vi "Change Language.vi"(9 "Array IN":string[][](array[string]), 10 "References Pane":T1(array[cluster]), 11 "Langues/Languages":u8) -> ()   [LabVIEW 2013]
doc: "Jean-Marc Simard \nExaprom inc. 2009"
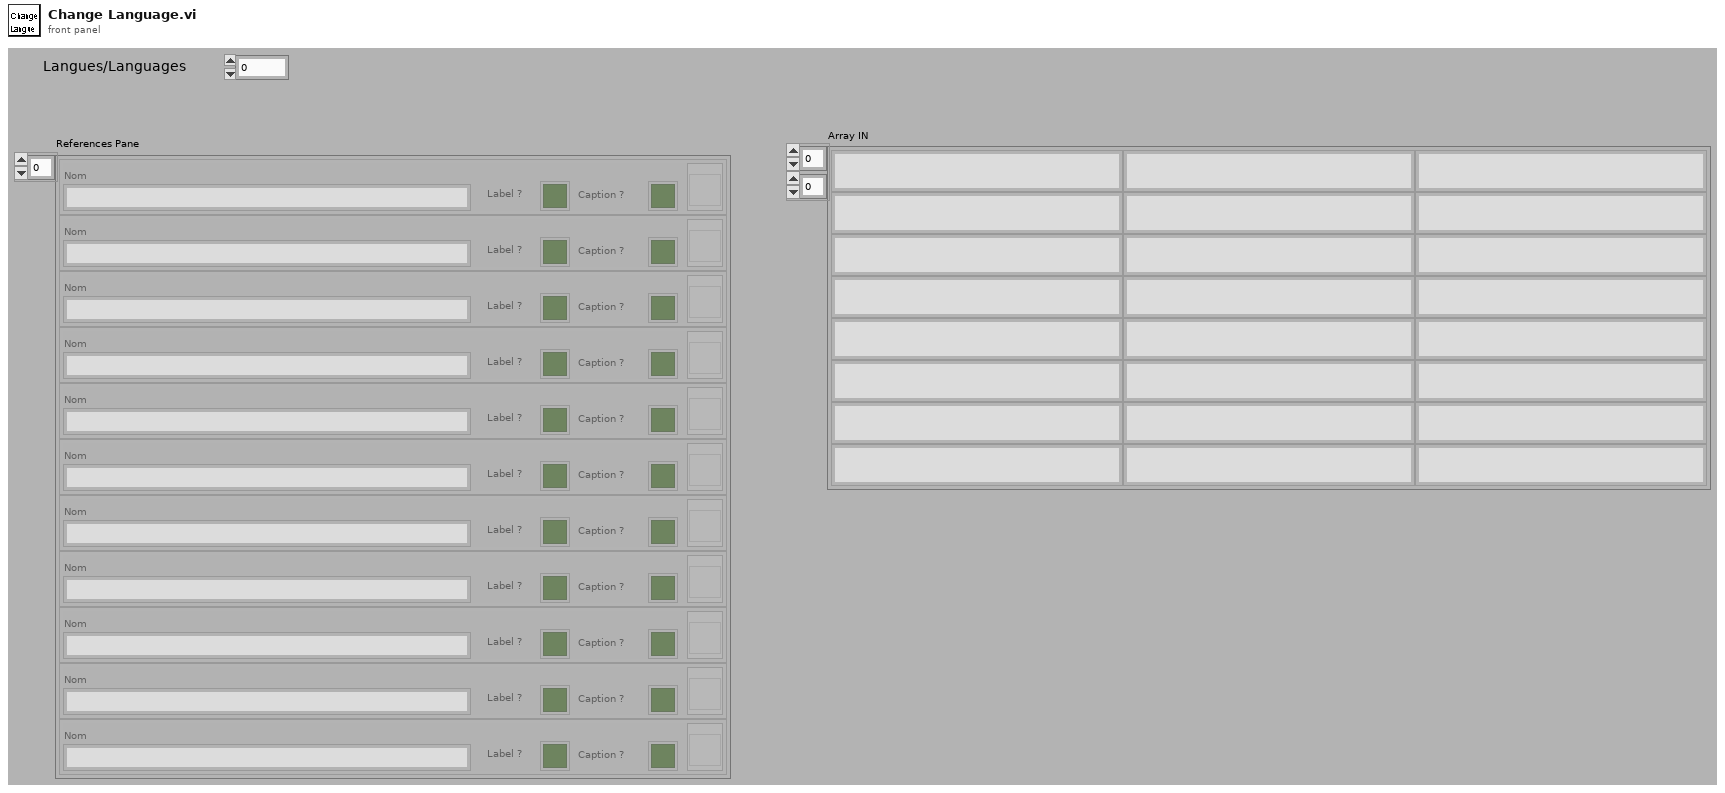
[diagram p1: front panel]
types:
  T1 = cluster{"Nom":string, "Label ?":bool, "Caption ?":bool, "Ref":refnum<vi>}[]
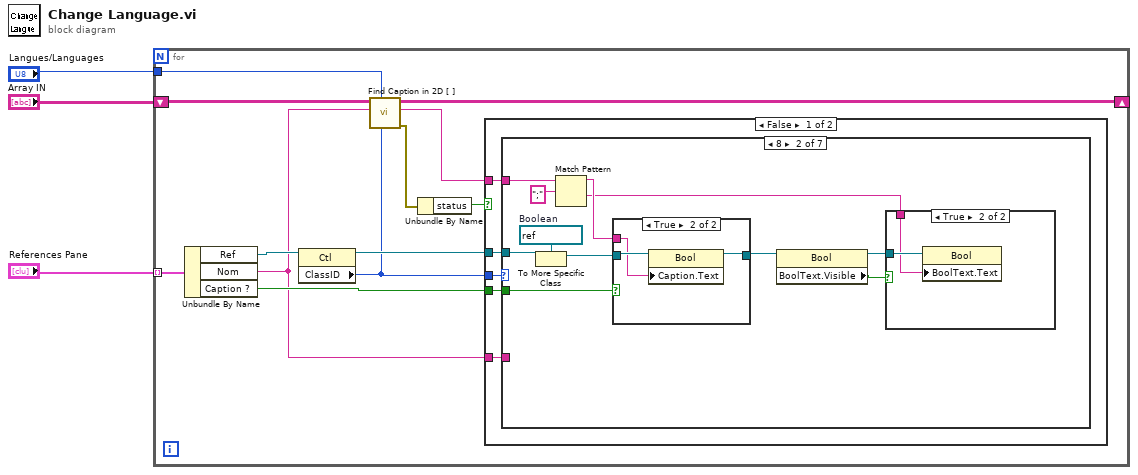
[diagram p0: block diagram]
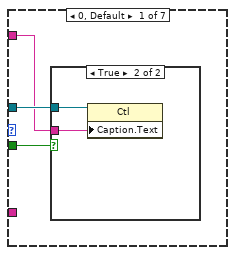
[diagram p2: hidden frame]
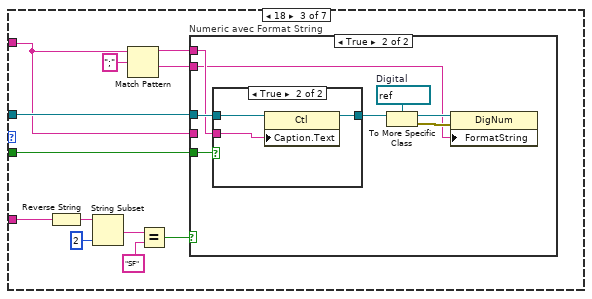
[diagram p6: hidden frame]
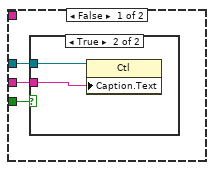
[diagram p7: hidden frame]
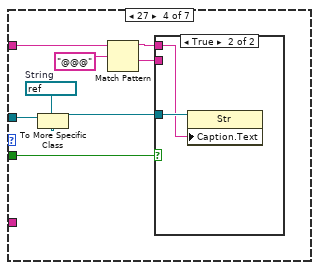
[diagram p10: hidden frame]
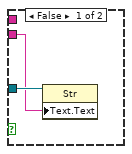
[diagram p11: hidden frame]
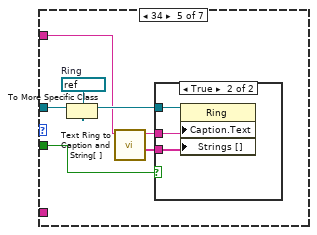
[diagram p12: hidden frame]
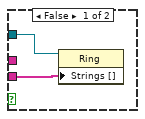
[diagram p13: hidden frame]
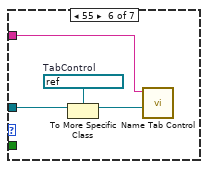
[diagram p14: hidden frame]
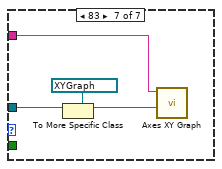
[diagram p15: hidden frame]
diagram:
  n1 = for {
    tunnel: "References Pane" -> [w5] mode=indexing
    shift-right: [w13] -> _
    shift-left: "Array IN" -> [w14]
    tunnel: "Langues/Languages" -> [w6]
    n2 = Unbundle By Name(w5) -> ("Ref"=w15:refnum<vi>, "Nom"=w4:string, "Caption ?"=w9:bool)
    n3 = property class="Ctl"(reference=w15) -> (reference out=w10:refnum<vi>, "ClassID"=w8:u32)  [unwired: 1 in, 1 out]
    n4 = call "Find Caption in 2D [ ].vi"("Class ID"=w8, "Langues/Languages"=w6, "Nom"=w4, "Array IN"=w14) -> ("error out"=w12:errorcluster, "Légende"=w11:string, "Array OUT"=w13:string[][])  [unwired: 1 in, 4 out]
    n5 = Unbundle By Name(w12) -> ("status"=w7:bool)
    n6 = case shown="False" w7 {
      tunnel: w10 -> [w20 _]
      tunnel: w11 -> [w19 _]
      tunnel: w8 -> [w18 _]
      tunnel: w9 -> [w17 _]
      tunnel: w4 -> [w16 _]
      frame False {
        n7 = case shown="8" w18 {
          tunnel: w20 -> [w23 w36 w49 w78 w89 w98 w102]
          tunnel: w19 -> [w22 w33 w46 w75 w86 w99 w103]
          tunnel: w17 -> [w21 w32 w48 w76 w87 _ _]
          tunnel: w16 -> [_ _ w43 _ _ _ _]
          frame 0, Default {
            n8 = case shown="True" w21 {
              tunnel: w23 -> [_ w25]
              tunnel: w22 -> [_ w24]
              frame False {
              }
              frame True {
                n9 = property class="Ctl"(reference=w25, "Caption.Text"=w24) -> ()  [unwired: 1 in, 2 out]
              }
            }
          }
          frame 8 {
            w35 = refnum<vi> refnum  # Boolean
            n10 = To More Specific Class(target class=w35, reference=w36) -> (specific class reference=w30:refnum<vi>)  [unwired: 1 in, 1 out]
            n11 = Match Pattern(string=w33, regular expression=";") -> (before substring=w31:string, after substring=w26:string)  [unwired: 3 out]
            n12 = case shown="True" w32 {
              tunnel: w31 -> [_ w41]
              tunnel: w30 -> [w39 w42]
              tunnel: [w39 w40] -> w29
              frame False {
              }
              frame True {
                n13 = property class="Bool"(reference=w42, "Caption.Text"=w41) -> (reference out=w40:refnum<vi>)  [unwired: 1 in, 1 out]
              }
            }
            n14 = property class="Bool"(reference=w29) -> (reference out=w27:refnum<vi>, "BoolText.Visible"=w28:bool)  [unwired: 1 in, 1 out]
            n15 = case shown="True" w28 {
              tunnel: w27 -> [_ w38]
              tunnel: w26 -> [_ w37]
              frame False {
              }
              frame True {
                n16 = property class="Bool"(reference=w38, "BoolText.Text"=w37) -> ()  [unwired: 1 in, 2 out]
              }
            }
          }
          frame 18 {
            n17 = Reverse String(1:w43) -> (0:w54:string)
            n18 = String Subset(string=w54, length (rest)=2 ("length (rest)")) -> (substring=w52:string)  [unwired: 1 out]
            n19 = Match Pattern(string=w46, regular expression=";") -> (before substring=w45:string, after substring=w44:string)  [unwired: 3 out]
            n20 = Equal?(x=w52, y="SF") -> (x = y?=w50:bool)
            n21 = case "Numeric avec Format String" shown="True" w50 {
              tunnel: w49 -> [w57 w67]
              tunnel: w46 -> [w56 _]
              tunnel: w48 -> [w55 w66]
              tunnel: w45 -> [_ w65]
              tunnel: w44 -> [_ w60]
              frame False {
                n22 = case shown="True" w55 {
                  tunnel: w57 -> [_ w59]
                  tunnel: w56 -> [_ w58]
                  frame False {
                  }
                  frame True {
                    n23 = property class="Ctl"(reference=w59, "Caption.Text"=w58) -> ()  [unwired: 1 in, 2 out]
                  }
                }
              }
              frame True {
                w61 = refnum<vi> refnum  # Digital
                n24 = case shown="True" w66 {
                  tunnel: w67 -> [w68 w71]
                  tunnel: w65 -> [_ w70]
                  tunnel: [w68 w69] -> w62
                  frame False {
                  }
                  frame True {
                    n25 = property class="Ctl"(reference=w71, "Caption.Text"=w70) -> (reference out=w69:refnum<vi>)  [unwired: 1 in, 1 out]
                  }
                }
                n26 = To More Specific Class(target class=w61, reference=w62) -> (specific class reference=w63:refnum<vi>, error out=w64:errorcluster)  [unwired: 1 in]
                n27 = property class="DigNum"(reference=w63, error in=w64, "FormatString"=w60) -> ()  [unwired: 2 out]
              }
            }
          }
          frame 27 {
            w79 = refnum<vi> refnum  # String
            n28 = To More Specific Class(target class=w79, reference=w78) -> (specific class reference=w77:refnum<vi>)  [unwired: 1 in, 1 out]
            n29 = Match Pattern(string=w75, regular expression="@@@") -> (before substring=w72:string, after substring=w73:string)  [unwired: 3 out]
            n30 = case shown="True" w76 {
              tunnel: w77 -> [w81 w83]
              tunnel: w73 -> [w80 _]
              tunnel: w72 -> [_ w82]
              frame False {
                n31 = property class="Str"(reference=w81, "Text.Text"=w80) -> ()  [unwired: 1 in, 2 out]
              }
              frame True {
                n32 = property class="Str"(reference=w83, "Caption.Text"=w82) -> ()  [unwired: 1 in, 2 out]
              }
            }
          }
          frame 34 {
            w90 = refnum<vi> refnum  # Ring
            n33 = To More Specific Class(target class=w90, reference=w89) -> (specific class reference=w88:refnum<vi>)  [unwired: 1 in, 1 out]
            n34 = call "Text Ring to Caption and String[ ].vi"("String"=w86) -> ("String[ ]"=w85:string[], "Caption"=w84:string)  [unwired: 1 in, 8 out]
            n35 = case shown="True" w87 {
              tunnel: w88 -> [w92 w95]
              tunnel: w85 -> [w91 w93]
              tunnel: w84 -> [_ w94]
              frame False {
                n36 = property class="Ring"(reference=w92, "Strings []"=w91) -> ()  [unwired: 1 in, 2 out]
              }
              frame True {
                n37 = property class="Ring"(reference=w95, "Caption.Text"=w94, "Strings []"=w93) -> ()  [unwired: 1 in, 2 out]
              }
            }
          }
          frame 55 {
            w96 = refnum<vi> refnum  # TabControl
            n38 = To More Specific Class(target class=w96, reference=w98) -> (specific class reference=w97:refnum<vi>)  [unwired: 1 in, 1 out]
            n39 = call "Name Tab Control.vi"("TabCtl Refnum"=w97, "String"=w99) -> ()  [unwired: 10 out]
          }
          frame 83 {
            n40 = To More Specific Class(target class=refnum<vi> refnum ("XYGraph Refnum"), reference=w102) -> (specific class reference=w101:refnum<vi>)  [unwired: 1 in, 1 out]
            n41 = call "Axes XY Graph.vi"("XYGraph Refnum"=w101, "String"=w103) -> ()  [unwired: 10 out]
          }
        }
      }
      frame True {
      }
    }
  }
